vi "SVT AC Induction Motor.vi"(0 "nominal speed [RPM]":dbl=3360.0, 1 "desired units":u16(ring) items=["Hz", "Order"], 5 "number of poles":u32=2, 7 "number of bars":u32=38, 9 "line frequency [Hz]":dbl=60.0, 11 "error in (no error)":errorcluster) -> (3 "synchronous speed [RPM]":dbl=3600.0, 4 "slip frequency":dbl=4.0, 6 "pole pass frequency":dbl=8.0, 8 "rotor bar pass frequency":dbl=2128.0, 15 "error out":errorcluster)   [LabVIEW 2017, in "SoundVib_MachineCharacteristic.lvlib"]
doc: "Calculates characteristic frequencies or orders of motors. You must manually select the polymorphic instance you want to use."
uses:
  <vilib>/addons/Sound and Vibration/svt_Machine Characteristic/SoundVib_MachineCharacteristic.lvlib
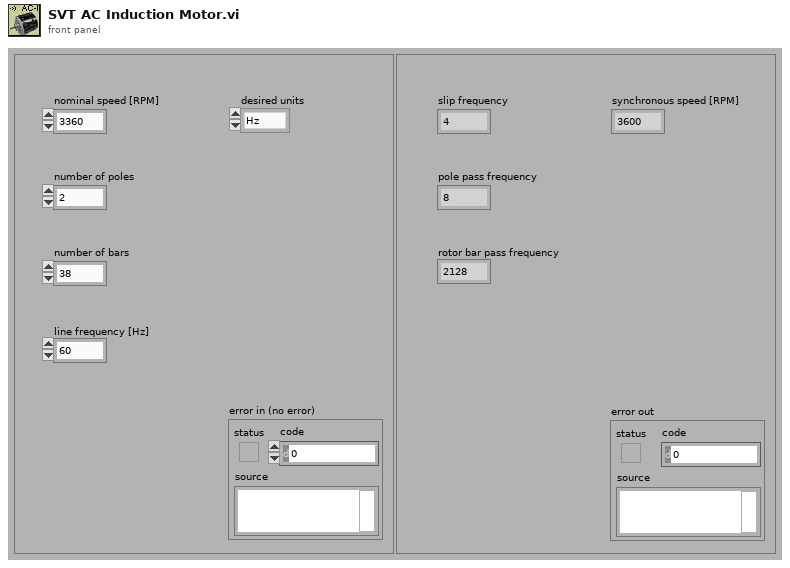
[diagram p1: front panel]
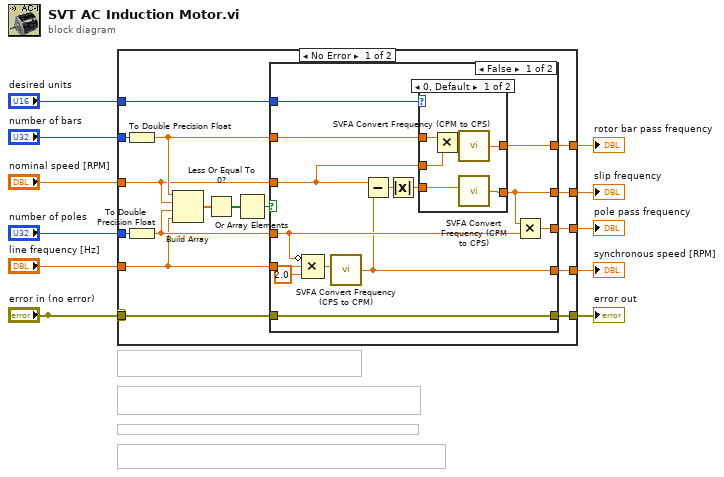
[diagram p0: block diagram]
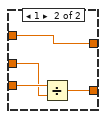
[diagram p2: hidden frame]
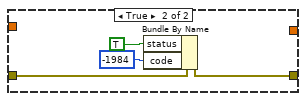
[diagram p3: hidden frame]
diagram:
  n1 = case shown="No Error" "error in (no error)" {
    selector: "error in (no error)" -> [_ w56]
    tunnel: [w21 w56] -> w11
    tunnel: "desired units" -> [w27 _]
    tunnel: "line frequency [Hz]" -> [w15 _]
    tunnel: "number of poles" -> [w19 _]
    tunnel: [w26 _] -> w7
    tunnel: "nominal speed [RPM]" -> [w17 _]
    tunnel: [w25 _] -> w5
    tunnel: [w24 _] -> w4
    tunnel: "number of bars" -> [w20 _]
    tunnel: [w23 _] -> w2
    tunnel: "error in (no error)" -> [w22 _]
    frame No Error {
      n2 = To Double Precision Float(number=w20) -> (double precision float=w18:dbl)
      n3 = To Double Precision Float(number=w19) -> (double precision float=w16:dbl)
      n4 = Build Array(w18, w17, w16, w15) -> (w14:dbl[])
      n5 = Less Or Equal To 0?(x=w14) -> (x <= 0?=w13:bool[])
      n6 = Or Array Elements(Boolean array=w13) -> (logical OR=w12:bool)
      n7 = case shown="False" w12 {
        tunnel: w27 -> [w41 _]
        tunnel: [w28 _] -> w26
        tunnel: [w33 _] -> w25
        tunnel: [w32 _] -> w24
        tunnel: [w38 _] -> w23
        tunnel: w17 -> [w37 _]
        tunnel: w15 -> [w36 _]
        tunnel: w22 -> [w35 w55]
        tunnel: [w35 w54] -> w21
        tunnel: w18 -> [w31 _]
        tunnel: w16 -> [w30 _]
        frame False {
          n8 = Compound Arithmetic op=MULTIPLY(invert w30, w36, 2.0 ("value")) -> (w29:dbl)
          n9 = call <vilib>:"SVFA Convert Frequency (CPS to CPM).vi"("frequency [Hz]"=w29) -> ("nominal [RPM]"=w28:dbl)  [unwired: 5 in]
          n10 = Subtract(x=w37, y=w28) -> (x-y=w39:dbl)
          n11 = Absolute Value(x=w39) -> (abs(x)=w34:dbl)
          n12 = case shown="0, Default" w41 {
            tunnel: w34 -> [w43 w51]
            tunnel: [w42 w49] -> w33
            tunnel: [w44 w48] -> w38
            tunnel: w37 -> [w46 w50]
            tunnel: w31 -> [w47 w48]
            frame 0, Default {
              n13 = Multiply(x=w47, y=w46) -> (x*y=w45:dbl)
              n14 = call <vilib>:"SVFA Convert Frequency (CPM to CPS).vi"("nominal speed [RPM]"=w45) -> ("frequency [Hz]"=w44:dbl)  [unwired: 5 in]
              n15 = call <vilib>:"SVFA Convert Frequency (CPM to CPS).vi"("nominal speed [RPM]"=w43) -> ("frequency [Hz]"=w42:dbl)  [unwired: 5 in]
            }
            frame 1 {
              n16 = Divide(x=w51, y=w50) -> (x/y=w49:dbl)
            }
          }
          n17 = Multiply(x=w33, y=w30) -> (x*y=w32:dbl)
        }
        frame True {
          n18 = Bundle By Name(cluster=w55, "status"=TRUE, "code"=-1984) -> (w54:errorcluster)
        }
      }
    }
    frame Error {
    }
  }
  "rotor bar pass frequency" <- w2
  "pole pass frequency" <- w4
  "slip frequency" <- w5
  "synchronous speed [RPM]" <- w7
  "error out" <- w11
